vi "LoadingTunedData.vi"(0 "Refnum in":refnum<visa-resource-name>, 1 "Mode":T1, 3 "error in (no error)":errorcluster, 4 "StartAddr":i32) -> (9 "INT":i32[](array[numeric]), 10 "error out":errorcluster)   [LabVIEW 2020]
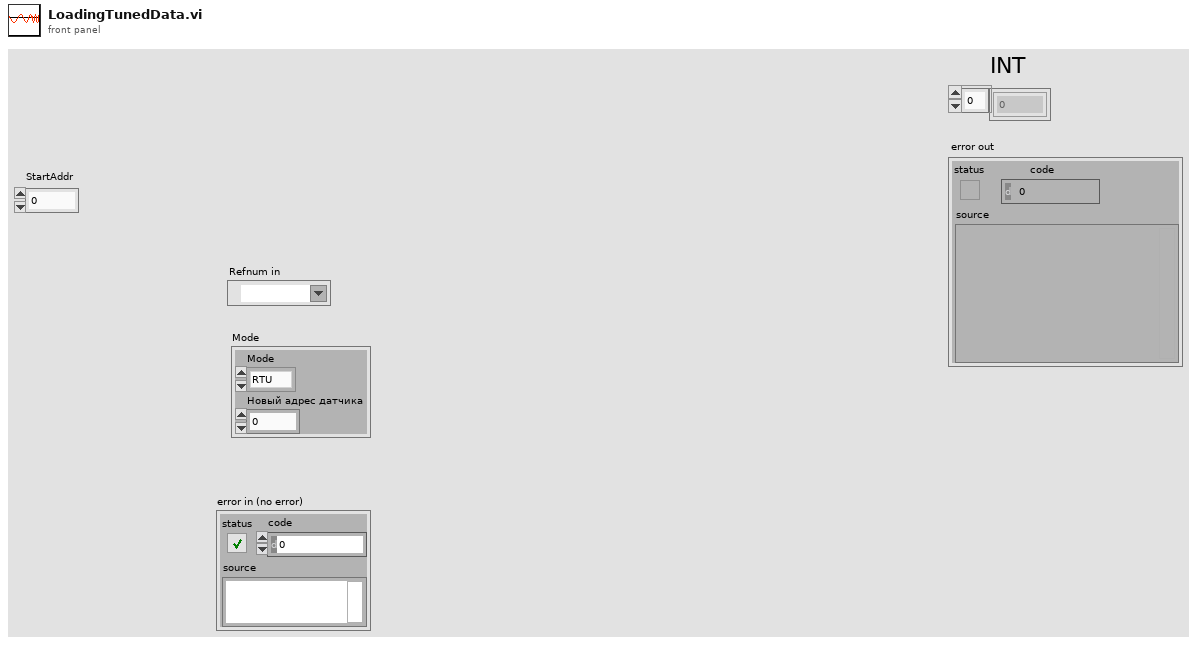
[diagram p1: front panel]
types:
  T1 = cluster{"Mode":enum16{"RTU", "ASCII"}, "Новый адрес датчика":u16}
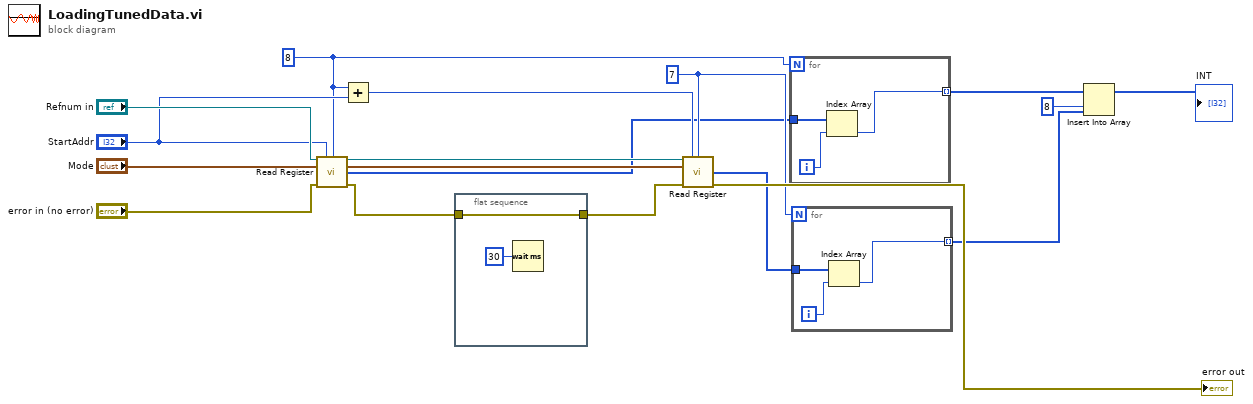
[diagram p0: block diagram]
diagram:
  w3 = 7
  w9 = 8
  n1 = call "Read Register.vi"("Refnum in"="Refnum in", "startReg"="StartAddr", "Quantity"=w9, "Mode"="Mode", "error in (no error)"="error in (no error)") -> ("Refnum Out"=w15:refnum<visa-resource-name>, "ModeOut"=w14:T1, "Holding Registers"=w1:u16[], "error out"=w13:errorcluster)  [unwired: 6 in, 1 out]
  n2 = Add(x=w9, y="StartAddr") -> (x+y=w10:i32)
  n3 = flat-sequence {
    tunnel: w13 -> [w20]
    tunnel: [w20] -> w12
    frame #0 {
      n4 = Wait (ms)(milliseconds to wait=u32 30) -> ()  [unwired: 1 out]
    }
  }
  n5 = call "Read Register.vi"("Refnum in"=w15, "startReg"=w10, "Quantity"=w3, "Mode"=w14, "error in (no error)"=w12) -> ("Holding Registers"=w2:u16[], "error out"=→"error out":errorcluster)  [unwired: 6 in, 3 out]
  n6 = for {
    N: w9 -> [_]
    tunnel: w1 -> [w23]
    tunnel: [w21] -> w7 mode=indexing
    i -> [w22]
    n7 = Index Array(array=w23, index=w22) -> (element=w21:u16)
  }
  n8 = for {
    N: w3 -> [_]
    tunnel: w2 -> [w26]
    tunnel: [w24] -> w5 mode=indexing
    i -> [w25]
    n9 = Index Array(array=w26, index=w25) -> (element=w24:u16)
  }
  n10 = Insert Into Array(array=w7, index=8, new element=w5) -> (→"INT":u16[])
